vi "DAQ_trigger_AOTF_with_camera_fire.vi"(0 "Analogic output":tag, 1 "Time resolution (s)":dbl=1e-05, 2 "Start.Retriggerable":bool, 3 "Initial phase shift (s)":dbl=0.001, 5 "Trigger source":tag, 7 "Pulse intensity (V)":dbl=1.0 format="%#_6p", 9 "counter":tag, 11 "error in":errorcluster, 12 "Pulse length Ton (s)":dbl=0.025, 14 "Pulse length Toff (s)":dbl=0.01) -> (4 "AOTF trigger task":refnum<k21>, 10 "counter task":refnum<k21>, 15 "error out":errorcluster)   [LabVIEW 2015]
uses:
  <vilib>/DAQmx/write.llb/DAQmx Write (Analog Wfm 1Chan NSamp).vi
  <vilib>/DAQmx/create/channels.llb/DAQmx Create Channel (AO-Voltage-Basic).vi
  <vilib>/DAQmx/create/channels.llb/DAQmx Create Channel (CO-Pulse Generation-Frequency).vi
  <vilib>/DAQmx/configure/timing.llb/DAQmx Timing (Implicit).vi
  <vilib>/DAQmx/configure/timing.llb/DAQmx Timing (Sample Clock).vi
  <vilib>/DAQmx/configure/trigger.llb/DAQmx Start Trigger (Digital Edge).vi
  <vilib>/DAQmx/miscellaneous.llb/DAQmx Fill In Error Info.vi
  <resource>/objmgr/daqmx.rc
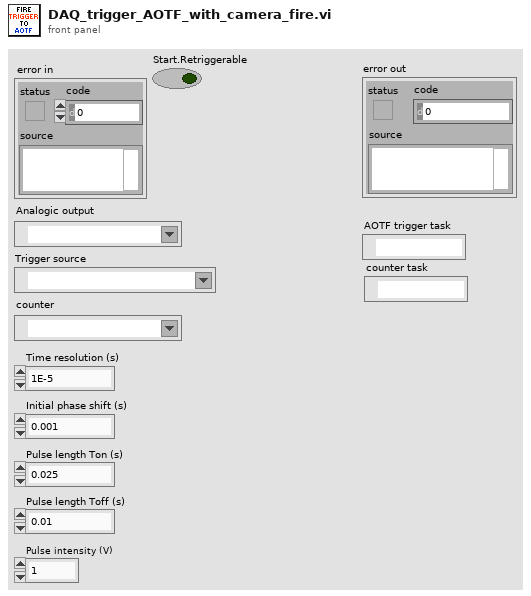
[diagram p1: front panel]
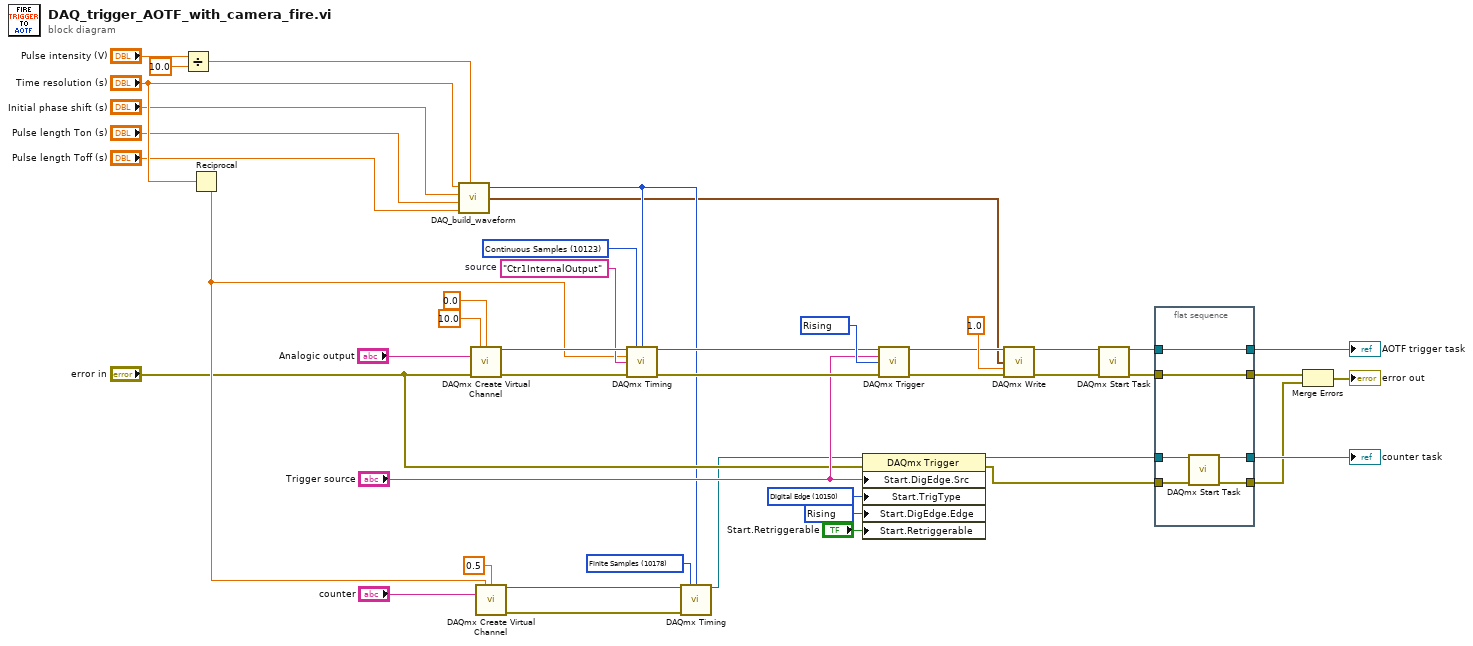
[diagram p0: block diagram]
diagram:
  w12 = "Ctr1InternalOutput"  # source
  w23 = 10178 items=["Finite Samples"=10178, "Continuous Samples"=10123, "Hardware Timed Single Point"=12522] ("sample mode")
  w31 = 10280 items=["Rising"=10280, "Falling"=10171] ("Start.DigEdge.Edge")
  w32 = 10150 items=["Analog Edge"=10099, "Digital Edge"=10150, "Digital Pattern"=10398, "Analog Window"=10103, "None"=10230] ("Start.TrigType")
  w39 = 10280 items=["Rising"=10280, "Falling"=10171] ("edge")
  w41 = 10123 items=["Finite Samples"=10178, "Continuous Samples"=10123, "Hardware Timed Single Point"=12522] ("sample mode")
  n1 = Divide(x="Pulse intensity (V)", y=10.0) -> (x/y=w14:dbl)
  n2 = Reciprocal(x="Time resolution (s)") -> (1/x=w6:dbl)
  n3 = call "DAQ_build_waveform.vi"("Résolution temporelle"="Time resolution (s)", "Décalage"="Initial phase shift (s)", "Largeur impulsion"="Pulse length Ton (s)", "Remise à 0"="Pulse length Toff (s)", "Pulse intensity"=w14) -> ("size(s)"=w4:i32, "waveform"=w3:waveform(dbl))  [unwired: 1 out]
  n4 = call-poly <vilib>:"DAQmx Create Virtual Channel.vi"("maximum value"=10.0, "minimum value"=0.0, "physical channels"="Analogic output", "error in"="error in") -> ("task out"=w42:refnum<k21>, "error out"=w40:errorcluster)  [unwired: 10 in]
  n5 = call-poly <vilib>:"DAQmx Create Virtual Channel.vi"("frequency"=w6, "duty cycle"=0.5, "counter"="counter") -> ("task out"=w25:refnum<k21>, "error out"=w24:errorcluster)  [unwired: 11 in]
  n6 = call-poly <vilib>:"DAQmx Timing.vi"("task/channels in"=w42, "sample mode"=w41, "samples per channel"=w4, "rate"=w6, "source"=w12, "error in"=w40) -> ("task out"=w37:refnum<k21>, "error out"=w38:errorcluster)  [unwired: 8 in]
  n7 = call-poly <vilib>:"DAQmx Timing.vi"("task/channels in"=w25, "sample mode"=w23, "samples per channel"=w4, "error in"=w24) -> ("task out"=w2:refnum<k21>)  [unwired: 10 in, 1 out]
  n8 = property class="DAQmx Trigger"(reference=w2, error in="error in", "Start.DigEdge.Src"="Trigger source", "Start.TrigType"=w32, "Start.DigEdge.Edge"=w31, "Start.Retriggerable"="Start.Retriggerable") -> (reference out=w29:refnum<k21>, error out=w28:errorcluster)
  n9 = call-poly <vilib>:"DAQmx Trigger.vi"("task/channels in"=w37, "source"="Trigger source", "edge"=w39, "error in"=w38) -> ("task out"=w16:refnum<k21>, "error out"=w36:errorcluster)  [unwired: 10 in]
  n10 = call-poly <vilib>:"DAQmx Write.vi"("task/channels in"=w16, "data"=w3, "timeout"=1.0, "error in"=w36) -> ("task out"=w34:refnum<k21>, "error out"=w33:errorcluster)  [unwired: 9 in, 1 out]
  n11 = call <vilib>:"DAQmx Start Task.vi"("task/channels in"=w34, "error in"=w33) -> ("task out"=w22:refnum<k21>, "error out"=w30:errorcluster)  [unwired: 12 in]
  n12 = flat-sequence {
    tunnel: w30 -> [w48]
    tunnel: w29 -> [w51]
    tunnel: w28 -> [w50]
    tunnel: [w49] -> w17
    tunnel: [w48] -> w18
    tunnel: [w47] -> w45
    tunnel: w22 -> [w47]
    tunnel: [w46] -> w44
    frame #0 {
      n13 = call <vilib>:"DAQmx Start Task.vi"("task/channels in"=w51, "error in"=w50) -> ("task out"=w46:refnum<k21>, "error out"=w49:errorcluster)  [unwired: 12 in]
    }
  }
  n14 = Merge Errors(w18, w17) -> (→"error out":errorcluster)
  "AOTF trigger task" <- w45
  "counter task" <- w44
